vi "Новая проверка Витерби.vi"() -> ()   [LabVIEW 2013]
uses:
  IS-95/transmitter/9600/syndrom(9600).vi
  IS-95/receiver/common/metrics.vi
  <vilib>/ptbypt/NI_PtbyPt.lvlib
panel:
  out "frame/sec":dbl
  out "Numeric":i32
  out "Pb":dbl
  in  "ОСШ(дБ)":dbl(knob)=3.0121235001212314 scale=0.0..10.0
  in  "stop":bool
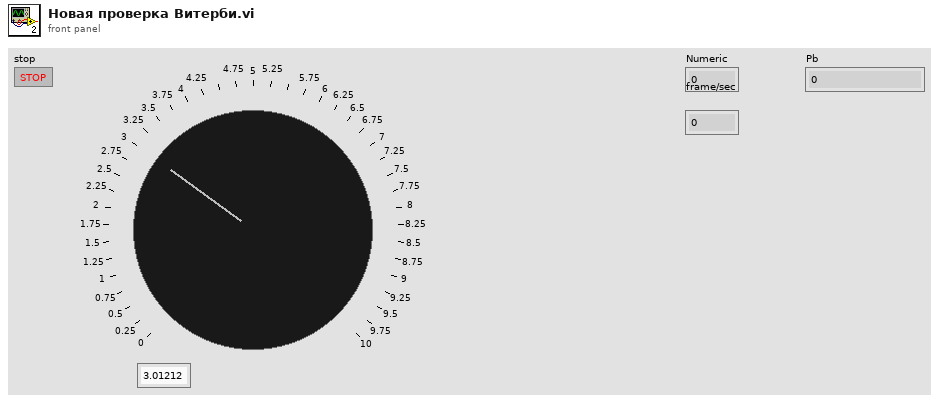
[diagram p1: front panel]
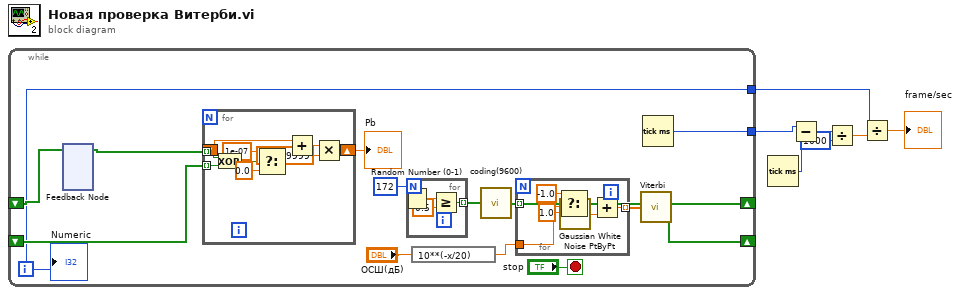
[diagram p0: block diagram]
diagram:
  n1 = while {
    shift-right: [w14] -> _
    shift-left: _ -> [w11]
    shift-right: [w13] -> _
    shift-left: _ -> [w12]
    tunnel: [w9] -> w7
    tunnel: [w8] -> w2
    i -> [w8]
    stop <- "stop" stop-if-true
    n2 = feedback #1() -> (w10:bool[])  [unwired: 1 in]
    n3 = feedback-in #1(w11) -> ()
    n4 = for {
      tunnel: w12 -> [w26] mode=indexing
      tunnel: w10 -> [w24] mode=indexing
      shift-right: [w23] -> w15
      shift-left: _ -> [w22]
      n5 = Exclusive Or(1:w26, 2:w24) -> (0:w31:bool)
      n6 = Select(t=1e-07, s=w31, f=0.0) -> (s? t:f=w29:dbl)
      n7 = Add(x=w22, y=w29) -> (x+y=w28:dbl)
      n8 = Multiply(x=w28, y=0.9999999) -> (x*y=w23:dbl)
    }
    "Pb" <- w15
    n9 = for {
      N: 172 -> [_]
      tunnel: [w39] -> w16 mode=indexing
      n10 = Random Number (0-1)() -> (number: 0 to 1=w41:dbl)
      n11 = Greater Or Equal?(x=w41, y=0.5) -> (x >= y?=w39:bool)
    }
    n12 = expression code="10**(-x/20)"("ОСШ(дБ)") -> (w18:dbl)
    n13 = call "coding(9600).vi"("Кадр на вход\nкодера"=w16) -> ("Поток кодированных \nбитов"=w14:bool[])  [unwired: 14 in]
    n14 = for {
      tunnel: w14 -> [w38] mode=indexing
      tunnel: [w33] -> w19 mode=indexing
      tunnel: w18 -> [w32]
      n15 = Select(t=-1.0, s=w38, f=1.0) -> (s? t:f=w35:dbl)
      n16 = call <vilib>:"Gaussian White Noise PtByPt.vi"("standard deviation"=w32) -> ("Gaussian white noise"=w34:dbl)  [unwired: 2 in]
      n17 = Add(x=w35, y=w34) -> (x+y=w33:dbl)
    }
    n18 = call "Viterbi.vi"("Кадр с мягкими\nзначениями"=w19) -> ("Декодированный поток битов"=w13:bool[])  [unwired: 14 in]
    n19 = Tick Count (ms)() -> (millisecond timer value=w9:u32)
    "Numeric" <- w8
  }
  n20 = Tick Count (ms)() -> (millisecond timer value=w6:u32)
  n21 = Subtract(x=w7, y=w6) -> (x-y=w5:u32)
  n22 = Divide(x=w5, y=u32 1000) -> (x/y=w3:dbl)
  n23 = Divide(x=w2, y=w3) -> (x/y=→"frame/sec":dbl)
